vi "TherapyInfo.vi"(0 "refnum":refnum<file>, 11 "offset":i32) -> (3 "Therapy Parameters":T1 {"Therapy amplitude (mV)" min=50 max=1000 format="%.2f"; "Time on (s)" format="%.3f"; "Theraputic Freq (MHz)" format="%.3f"}, 4 "dup refnum":refnum<file>, 6 "Theraputic Freq (MHz)":sgl=0.1 format="%.3f", 8 "Time on (s)":sgl=1.0 format="%.3f", 10 "Therapy amplitude (mV)":sgl=50.0 min=50 max=1000 format="%.2f", 15 "Lines Before":u16=20)   [LabVIEW 2022 SP3]
panel:
  out "Lines After":u16=80
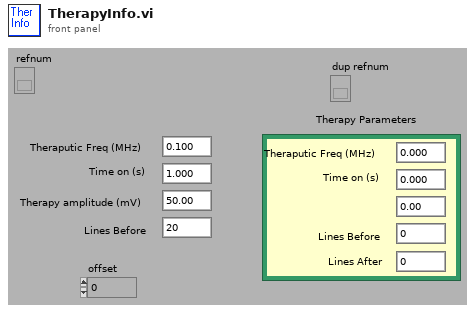
[diagram p1: front panel]
types:
  T1 = cluster{"Theraputic Freq (MHz)":sgl, "Time on (s)":sgl, "Therapy amplitude (mV)":sgl, "Lines Before":u16, "Lines After":u16}
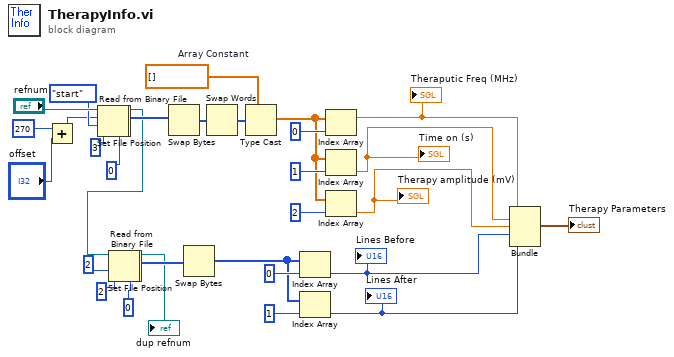
[diagram p0: block diagram]
diagram:
  w16 = sgl[] []  # Array Constant
  n1 = Add(x=270 ("pos offset (0)"), y="offset") -> (x+y=w6:i32)
  n2 = Set File Position(offset (in bytes) (0)=w6, refnum="refnum", from (0:start)=enum16{"start", "end", "current"}."start" ("pos mode (0:2)")) -> (refnum out=w2:refnum<file>, error out=w1:errorcluster)  [unwired: 1 in]
  n3 = Read from Binary File(5:0, 8:w1, 10:3 ("count"), 11:w2) -> (2:w17:i32[], 3:w11:refnum<file>)  [unwired: 4 out]
  n4 = Set File Position(refnum=w11, from (0:start)=2) -> (refnum out=w4:refnum<file>, error out=w3:errorcluster)  [unwired: 1 in, 1 out]
  n5 = Read from Binary File(5:u16 0, 8:w3, 10:2 ("count"), 11:w4) -> (2:w22:u16[], 3:→"dup refnum":refnum<file>)  [unwired: 4 out]
  n6 = Swap Bytes(anything=w17) -> (byte swapped=w25:i32[])
  n7 = Swap Bytes(anything=w22) -> (byte swapped=w19:u16[])
  n8 = Swap Words(1:w25) -> (0:w24:i32[])
  n9 = Type Cast(type=w16, x=w24) -> (*(type *) &x=w15:sgl[])
  n10 = Index Array(array=w19, index=0) -> (element=w9:u16)
  "Lines Before" <- w9
  n11 = Index Array(array=w19, index=1) -> (element=w8:u16)
  "Lines After" <- w8
  n12 = Index Array(array=w15, index=0) -> (element=w14:sgl)
  "Theraputic Freq (MHz)" <- w14
  n13 = Index Array(array=w15, index=1) -> (element=w13:sgl)
  "Time on (s)" <- w13
  n14 = Index Array(array=w15, index=2) -> (element=w12:sgl)
  "Therapy amplitude (mV)" <- w12
  n15 = Bundle(w14, w13, w12, w9, w8) -> (→"Therapy Parameters":cluster{sgl, sgl, sgl, u16, u16})  [unwired: 1 out]
